vi "FeedbackDecode.vi"() -> ()   [LabVIEW 2020] (continued)
                n758 = Concatenate Strings(w456, ";SS.ExcludeSE=0;" ("EventStr"), w448) -> (w453:string)
                n759 = call "FeedbackDecode_WriteTextEOL.vi"("text"=w453, "refnum in"=w454) -> ()  [unwired: 8 in, 2 out]
                n760 = Bundle By Name(cluster=w460, "EventStr"=w453) -> (w452:T5)
                n761 = call "FeedbackDecode_MLComCtrl.vi"("DecodeClustIn"=w452, "Mode"=T19."SendEvent") -> ()  [unwired: 6 in, 4 out]
              }
              frame True {
                n762 = local read "LoopCnt"() -> (w471:u64)
                n763 = local read "NIPTime"() -> (w465:dbl)
                n764 = Format Into String(w471) -> (resulting string=w461:string)  [unwired: 3 in, 1 out]
                n765 = Concatenate Strings("ExcludeSE:SS.EventID=" ("string"), w461) -> (w470:string)
                n766 = call-poly "FeedbackDecode_VariablesToString.vi"("Format"="%0.0f", "ValueIn"=w465, "FieldName"="NIPTime" ("Key Word")) -> ("StringOut"=w462:string)  [unwired: 4 in]
                n767 = local read "EventParamsFID"() -> (w468:refnum<file>)
                n768 = local read "DecodeClust"() -> (w474:T5)
                n769 = Concatenate Strings(w470, ";SS.ExcludeSE=1;" ("EventStr"), w462) -> (w467:string)
                n770 = call "FeedbackDecode_WriteTextEOL.vi"("text"=w467, "refnum in"=w468) -> ()  [unwired: 8 in, 2 out]
                n771 = Bundle By Name(cluster=w474, "EventStr"=w467) -> (w466:T5)
                n772 = call "FeedbackDecode_MLComCtrl.vi"("DecodeClustIn"=w466, "Mode"=T19."SendEvent") -> ()  [unwired: 6 in, 4 out]
              }
            }
          }
          event Value Change {
            n773 = event-data() -> ("NewVal"=w476:bool)  [unwired: 1 in, 5 out]
            n774 = case shown="True" w476 {
              frame False {
                n775 = local read "LoopCnt"() -> (w487:u64)
                n776 = local read "NIPTime"() -> (w481:dbl)
                n777 = Format Into String(w487) -> (resulting string=w477:string)  [unwired: 3 in, 1 out]
                n778 = Concatenate Strings("StopAcqCAR:SS.EventID=" ("string"), w477) -> (w486:string)
                n779 = local read "EventParamsFID"() -> (w484:refnum<file>)
                n780 = call-poly "FeedbackDecode_VariablesToString.vi"("Format"="%0.0f", "ValueIn"=w481, "FieldName"="NIPTime" ("Key Word")) -> ("StringOut"=w478:string)  [unwired: 4 in]
                n781 = local read "DecodeClust"() -> (w490:T5)
                n782 = Concatenate Strings(w486, ";SS.AcqCAR=0;" ("EventStr"), w478) -> (w483:string)
                n783 = call "FeedbackDecode_WriteTextEOL.vi"("text"=w483, "refnum in"=w484) -> ()  [unwired: 8 in, 2 out]
                n784 = Bundle By Name(cluster=w490, "EventStr"=w483) -> (w482:T5)
                n785 = call "FeedbackDecode_MLComCtrl.vi"("DecodeClustIn"=w482, "Mode"=T19."SendEvent") -> ()  [unwired: 6 in, 4 out]
              }
              frame True {
                n786 = local read "LoopCnt"() -> (w501:u64)
                n787 = local read "NIPTime"() -> (w495:dbl)
                n788 = Format Into String(w501) -> (resulting string=w491:string)  [unwired: 3 in, 1 out]
                n789 = call-poly "FeedbackDecode_VariablesToString.vi"("Format"="%0.0f", "ValueIn"=w495, "FieldName"="NIPTime" ("Key Word")) -> ("StringOut"=w492:string)  [unwired: 4 in]
                n790 = Concatenate Strings("StartAcqCAR:SS.EventID=" ("string"), w491) -> (w500:string)
                n791 = local read "EventParamsFID"() -> (w498:refnum<file>)
                n792 = local read "DecodeClust"() -> (w504:T5)
                n793 = Concatenate Strings(w500, ";SS.AcqCAR=1;" ("EventStr"), w492) -> (w497:string)
                n794 = call "FeedbackDecode_WriteTextEOL.vi"("text"=w497, "refnum in"=w498) -> ()  [unwired: 8 in, 2 out]
                n795 = Bundle By Name(cluster=w504, "EventStr"=w497) -> (w496:T5)
                n796 = call "FeedbackDecode_MLComCtrl.vi"("DecodeClustIn"=w496, "Mode"=T19."SendEvent") -> ()  [unwired: 6 in, 4 out]
              }
            }
          }
          event Value Change {
            n797 = event-data() -> ("NewVal"=w506:bool)  [unwired: 1 in, 5 out]
            n798 = case shown="True" w506 {
              frame False {
              }
              frame True {
                n799 = stacked-sequence {
                  frame #0 {
                    n800 = local read "DecodeClust"() -> (w524:T5)
                    n801 = call "FeedbackDecode_MLComCtrl.vi"("DecodeClustIn"=w524, "Mode"=T19."BuildKalmanStr") -> ("DecodeClustOut"=w523:T5)  [unwired: 6 in, 3 out]
                    n802 = Unbundle By Name(w523) -> ("EventStr"=w531:string, "KalmanType"=w512:T44, "KDFFile"=w516:string)
                    n803 = local read "LoopCnt"() -> (w527:u64)
                    n804 = local read "NIPTime"() -> (w521:dbl)
                    n805 = Format Into String(format string="%s", w512) -> (resulting string=w509:string)  [unwired: 2 in, 1 out]
                    n806 = Format Into String(w527) -> (resulting string=w507:string)  [unwired: 3 in, 1 out]
                    n807 = call-poly "FeedbackDecode_VariablesToString.vi"("ValueIn"=w516, "FieldName"="KDFFile") -> ("StringOut"=w515:string)  [unwired: 5 in]
                    n808 = call-poly "FeedbackDecode_VariablesToString.vi"("Format"="%0.0f", "ValueIn"=w521, "FieldName"="NIPTime" ("Key Word")) -> ("StringOut"=w514:string)  [unwired: 4 in]
                    n809 = Concatenate Strings("ApplyTraining:SS.EventID=" ("string"), w507) -> (w526:string)
                    n810 = Concatenate Strings(w526, ";", w531) -> (w518:string)
                    n811 = local read "EventParamsFID"() -> (w525:refnum<file>)
                    n812 = Bundle By Name(cluster=w523, "EventStr"=w518) -> (w522:T5)
                    n813 = Concatenate Strings(w518, "SS.DecodeType='" ("FieldName"), w509, "';" ("string"), w515, w514) -> (w513:string)
                    n814 = call "FeedbackDecode_WriteTextEOL.vi"("text"=w513, "refnum in"=w525) -> ()  [unwired: 8 in, 2 out]
                    n815 = call "FeedbackDecode_MLComCtrl.vi"("DecodeClustIn"=w522, "Mode"=T19."SendEvent") -> ()  [unwired: 6 in, 4 out]
                  }
                  frame #1 {
                    n816 = property on="KinSrc" class="Enum (strict)"("Val(Sgnl)"=enum16{"Off", "Training", "Decode", "COB"}."Decode" ("Value (Signaling)")) -> ()  [unwired: 2 in, 2 out]
                  }
                }
              }
            }
          }
          event Value Change {
            n817 = event-data() -> ("NewVal"=w534:bool)  [unwired: 1 in, 5 out]
            n818 = case shown="True" w534 {
              frame False {
                n819 = local read "LoopCnt"() -> (w546:u64)
                n820 = local read "NIPTime"() -> (w540:dbl)
                n821 = Format Into String(w546) -> (resulting string=w536:string)  [unwired: 3 in, 1 out]
                n822 = call-poly "FeedbackDecode_VariablesToString.vi"("Format"="%0.0f", "ValueIn"=w540, "FieldName"="NIPTime" ("Key Word")) -> ("StringOut"=w537:string)  [unwired: 4 in]
                n823 = Concatenate Strings("DisableBaseline:SS.EventID=" ("string"), w536) -> (w545:string)
                n824 = local read "EventParamsFID"() -> (w543:refnum<file>)
                n825 = local read "DecodeClust"() -> (w549:T5)
                n826 = Concatenate Strings(w545, ";SS.ApplyBaseline=0;" ("EventStr"), w537) -> (w542:string)
                n827 = call "FeedbackDecode_WriteTextEOL.vi"("text"=w542, "refnum in"=w543) -> ()  [unwired: 8 in, 2 out]
                n828 = Bundle By Name(cluster=w549, "EventStr"=w542) -> (w541:T5)
                n829 = call "FeedbackDecode_MLComCtrl.vi"("DecodeClustIn"=w541, "Mode"=T19."SendEvent") -> ()  [unwired: 6 in, 4 out]
              }
              frame True {
                n830 = local read "LoopCnt"() -> (w560:u64)
                n831 = local read "NIPTime"() -> (w554:dbl)
                n832 = Format Into String(w560) -> (resulting string=w550:string)  [unwired: 3 in, 1 out]
                n833 = Concatenate Strings("EnableBaseline:SS.EventID=" ("string"), w550) -> (w559:string)
                n834 = local read "EventParamsFID"() -> (w557:refnum<file>)
                n835 = call-poly "FeedbackDecode_VariablesToString.vi"("Format"="%0.0f", "ValueIn"=w554, "FieldName"="NIPTime" ("Key Word")) -> ("StringOut"=w551:string)  [unwired: 4 in]
                n836 = local read "DecodeClust"() -> (w563:T5)
                n837 = Concatenate Strings(w559, ";SS.ApplyBaseline=1;" ("EventStr"), w551) -> (w556:string)
                n838 = call "FeedbackDecode_WriteTextEOL.vi"("text"=w556, "refnum in"=w557) -> ()  [unwired: 8 in, 2 out]
                n839 = Bundle By Name(cluster=w563, "EventStr"=w556) -> (w555:T5)
                n840 = call "FeedbackDecode_MLComCtrl.vi"("DecodeClustIn"=w555, "Mode"=T19."SendEvent") -> ()  [unwired: 6 in, 4 out]
              }
            }
          }
          event Value Change {
            n841 = event-data() -> ("NewVal"=w564:bool)  [unwired: 1 in, 5 out]
            n842 = case shown="True" w564 {
              frame False {
                n843 = disable-structure shown="Disabled" {
                  frame Disabled {
                    n844 = local read "LoopCnt"() -> (w576:u64)
                    n845 = local read "NIPTime"() -> (w570:dbl)
                    n846 = Format Into String(w576) -> (resulting string=w566:string)  [unwired: 3 in, 1 out]
                    n847 = call-poly "FeedbackDecode_VariablesToString.vi"("Format"="%0.0f", "ValueIn"=w570, "FieldName"="NIPTime" ("Key Word")) -> ("StringOut"=w567:string)  [unwired: 4 in]
                    n848 = Concatenate Strings("DisableBaseline:SS.EventID=" ("string"), w566) -> (w575:string)
                    n849 = local read "EventParamsFID"() -> (w573:refnum<file>)
                    n850 = local read "DecodeClust"() -> (w579:T5)
                    n851 = Concatenate Strings(w575, ";SS.ApplyBaseline=0;" ("EventStr"), w567) -> (w572:string)
                    n852 = call "FeedbackDecode_WriteTextEOL.vi"("text"=w572, "refnum in"=w573) -> ()  [unwired: 8 in, 2 out]
                    n853 = Bundle By Name(cluster=w579, "EventStr"=w572) -> (w571:T5)
                    n854 = call "FeedbackDecode_MLComCtrl.vi"("DecodeClustIn"=w571, "Mode"=T19."SendEvent") -> ()  [unwired: 6 in, 4 out]
                  }
                  frame Enabled {
                  }
                }
              }
              frame True {
                n855 = local read "LoopCnt"() -> (w590:u64)
                n856 = local read "NIPTime"() -> (w584:dbl)
                n857 = Format Into String(w590) -> (resulting string=w580:string)  [unwired: 3 in, 1 out]
                n858 = Concatenate Strings("ExportTraining:SS.EventID=" ("string"), w580) -> (w589:string)
                n859 = local read "EventParamsFID"() -> (w587:refnum<file>)
                n860 = call-poly "FeedbackDecode_VariablesToString.vi"("Format"="%0.0f", "ValueIn"=w584, "FieldName"="NIPTime" ("Key Word")) -> ("StringOut"=w581:string)  [unwired: 4 in]
                n861 = local read "DecodeClust"() -> (w593:T5)
                n862 = Concatenate Strings(w589, ";SS.ExportTraining=1;" ("EventStr"), w581) -> (w586:string)
                n863 = call "FeedbackDecode_WriteTextEOL.vi"("text"=w586, "refnum in"=w587) -> ()  [unwired: 8 in, 2 out]
                n864 = Bundle By Name(cluster=w593, "EventStr"=w586) -> (w585:T5)
                n865 = call "FeedbackDecode_MLComCtrl.vi"("DecodeClustIn"=w585, "Mode"=T19."SendEvent") -> ()  [unwired: 6 in, 4 out]
              }
            }
          }
          event Value Change {
            n866 = event-data() -> ("NewVal"=w594:bool)  [unwired: 1 in, 5 out]
            n867 = case shown="True" w594 {
              frame False {
                n868 = local read "LoopCnt"() -> (w606:u64)
                n869 = local read "NIPTime"() -> (w600:dbl)
                n870 = Format Into String(w606) -> (resulting string=w596:string)  [unwired: 3 in, 1 out]
                n871 = call-poly "FeedbackDecode_VariablesToString.vi"("Format"="%0.0f", "ValueIn"=w600, "FieldName"="NIPTime" ("Key Word")) -> ("StringOut"=w597:string)  [unwired: 4 in]
                n872 = Concatenate Strings("LatchingFilter:SS.EventID=" ("string"), w596) -> (w605:string)
                n873 = local read "EventParamsFID"() -> (w603:refnum<file>)
                n874 = local read "DecodeClust"() -> (w609:T5)
                n875 = Concatenate Strings(w605, ";SS.LatchingFilter=0;" ("EventStr"), w597) -> (w602:string)
                n876 = call "FeedbackDecode_WriteTextEOL.vi"("text"=w602, "refnum in"=w603) -> ()  [unwired: 8 in, 2 out]
                n877 = Bundle By Name(cluster=w609, "EventStr"=w602) -> (w601:T5)
                n878 = call "FeedbackDecode_MLComCtrl.vi"("DecodeClustIn"=w601, "Mode"=T19."SendEvent") -> ()  [unwired: 6 in, 4 out]
              }
              frame True {
                n879 = local read "LoopCnt"() -> (w620:u64)
                n880 = local read "NIPTime"() -> (w614:dbl)
                n881 = Format Into String(w620) -> (resulting string=w610:string)  [unwired: 3 in, 1 out]
                n882 = Concatenate Strings("LatchingFilter:SS.EventID=" ("string"), w610) -> (w619:string)
                n883 = local read "EventParamsFID"() -> (w617:refnum<file>)
                n884 = call-poly "FeedbackDecode_VariablesToString.vi"("Format"="%0.0f", "ValueIn"=w614, "FieldName"="NIPTime" ("Key Word")) -> ("StringOut"=w611:string)  [unwired: 4 in]
                n885 = local read "DecodeClust"() -> (w623:T5)
                n886 = Concatenate Strings(w619, ";SS.LatchingFilter=1;" ("EventStr"), w611) -> (w616:string)
                n887 = call "FeedbackDecode_WriteTextEOL.vi"("text"=w616, "refnum in"=w617) -> ()  [unwired: 8 in, 2 out]
                n888 = Bundle By Name(cluster=w623, "EventStr"=w616) -> (w615:T5)
                n889 = call "FeedbackDecode_MLComCtrl.vi"("DecodeClustIn"=w615, "Mode"=T19."SendEvent") -> ()  [unwired: 6 in, 4 out]
              }
            }
          }
          event Value Change {
            n890 = event-data() -> ("NewVal"=w624:bool)  [unwired: 1 in, 5 out]
            n891 = case shown="True" w624 {
              frame False {
                n892 = local read "LoopCnt"() -> (w636:u64)
                n893 = local read "NIPTime"() -> (w630:dbl)
                n894 = Format Into String(w636) -> (resulting string=w626:string)  [unwired: 3 in, 1 out]
                n895 = call-poly "FeedbackDecode_VariablesToString.vi"("Format"="%0.0f", "ValueIn"=w630, "FieldName"="NIPTime" ("Key Word")) -> ("StringOut"=w627:string)  [unwired: 4 in]
                n896 = Concatenate Strings("EEGTrigger:SS.EventID=" ("string"), w626) -> (w635:string)
                n897 = local read "EventParamsFID"() -> (w633:refnum<file>)
                n898 = local read "DecodeClust"() -> (w639:T5)
                n899 = Concatenate Strings(w635, ";SS.EEGTrigger=0;" ("EventStr"), w627) -> (w632:string)
                n900 = call "FeedbackDecode_WriteTextEOL.vi"("text"=w632, "refnum in"=w633) -> ()  [unwired: 8 in, 2 out]
                n901 = Bundle By Name(cluster=w639, "EventStr"=w632) -> (w631:T5)
                n902 = call "FeedbackDecode_MLComCtrl.vi"("DecodeClustIn"=w631, "Mode"=T19."SendEvent") -> ()  [unwired: 6 in, 4 out]
              }
              frame True {
                n903 = local read "LoopCnt"() -> (w650:u64)
                n904 = local read "NIPTime"() -> (w644:dbl)
                n905 = Format Into String(w650) -> (resulting string=w640:string)  [unwired: 3 in, 1 out]
                n906 = Concatenate Strings("EEGTrigger:SS.EventID=" ("string"), w640) -> (w649:string)
                n907 = local read "EventParamsFID"() -> (w647:refnum<file>)
                n908 = call-poly "FeedbackDecode_VariablesToString.vi"("Format"="%0.0f", "ValueIn"=w644, "FieldName"="NIPTime" ("Key Word")) -> ("StringOut"=w641:string)  [unwired: 4 in]
                n909 = local read "DecodeClust"() -> (w653:T5)
                n910 = Concatenate Strings(w649, ";SS.EEGTrigger=1;" ("EventStr"), w641) -> (w646:string)
                n911 = call "FeedbackDecode_WriteTextEOL.vi"("text"=w646, "refnum in"=w647) -> ()  [unwired: 8 in, 2 out]
                n912 = Bundle By Name(cluster=w653, "EventStr"=w646) -> (w645:T5)
                n913 = call "FeedbackDecode_MLComCtrl.vi"("DecodeClustIn"=w645, "Mode"=T19."SendEvent") -> ()  [unwired: 6 in, 4 out]
              }
            }
          }
          event Value Change {
            n914 = event-data() -> ("NewVal"=w654:bool)  [unwired: 1 in, 5 out]
            n915 = case shown="True" w654 {
              frame False {
                n916 = local read "LoopCnt"() -> (w666:u64)
                n917 = local read "NIPTime"() -> (w660:dbl)
                n918 = Format Into String(w666) -> (resulting string=w656:string)  [unwired: 3 in, 1 out]
                n919 = call-poly "FeedbackDecode_VariablesToString.vi"("Format"="%0.0f", "ValueIn"=w660, "FieldName"="NIPTime" ("Key Word")) -> ("StringOut"=w657:string)  [unwired: 4 in]
                n920 = Concatenate Strings("ConnectECG:SS.EventID=" ("string"), w656) -> (w665:string)
                n921 = local read "EventParamsFID"() -> (w663:refnum<file>)
                n922 = local read "DecodeClust"() -> (w669:T5)
                n923 = Concatenate Strings(w665, ";SS.ConnectECG=0;" ("EventStr"), w657) -> (w662:string)
                n924 = call "FeedbackDecode_WriteTextEOL.vi"("text"=w662, "refnum in"=w663) -> ()  [unwired: 8 in, 2 out]
                n925 = Bundle By Name(cluster=w669, "EventStr"=w662) -> (w661:T5)
                n926 = call "FeedbackDecode_MLComCtrl.vi"("DecodeClustIn"=w661, "Mode"=T19."SendEvent") -> ()  [unwired: 6 in, 4 out]
              }
              frame True {
                n927 = local read "LoopCnt"() -> (w680:u64)
                n928 = local read "NIPTime"() -> (w674:dbl)
                n929 = Format Into String(w680) -> (resulting string=w670:string)  [unwired: 3 in, 1 out]
                n930 = Concatenate Strings("ConnectECG:SS.EventID=" ("string"), w670) -> (w679:string)
                n931 = local read "EventParamsFID"() -> (w677:refnum<file>)
                n932 = call-poly "FeedbackDecode_VariablesToString.vi"("Format"="%0.0f", "ValueIn"=w674, "FieldName"="NIPTime" ("Key Word")) -> ("StringOut"=w671:string)  [unwired: 4 in]
                n933 = local read "DecodeClust"() -> (w683:T5)
                n934 = Concatenate Strings(w679, ";SS.ConnectECG=1;" ("EventStr"), w671) -> (w676:string)
                n935 = call "FeedbackDecode_WriteTextEOL.vi"("text"=w676, "refnum in"=w677) -> ()  [unwired: 8 in, 2 out]
                n936 = Bundle By Name(cluster=w683, "EventStr"=w676) -> (w675:T5)
                n937 = call "FeedbackDecode_MLComCtrl.vi"("DecodeClustIn"=w675, "Mode"=T19."SendEvent") -> ()  [unwired: 6 in, 4 out]
              }
            }
          }
          event Value Change {
            n938 = event-data() -> ("NewVal"=w684:bool)  [unwired: 1 in, 5 out]
            n939 = case shown="False" w684 {
              frame False {
                n940 = local read "LoopCnt"() -> (w696:u64)
                n941 = local read "NIPTime"() -> (w690:dbl)
                n942 = Format Into String(w696) -> (resulting string=w686:string)  [unwired: 3 in, 1 out]
                n943 = call-poly "FeedbackDecode_VariablesToString.vi"("Format"="%0.0f", "ValueIn"=w690, "FieldName"="NIPTime" ("Key Word")) -> ("StringOut"=w687:string)  [unwired: 4 in]
                n944 = Concatenate Strings("ConnectIMU:SS.EventID=" ("string"), w686) -> (w695:string)
                n945 = local read "EventParamsFID"() -> (w693:refnum<file>)
                n946 = local read "DecodeClust"() -> (w699:T5)
                n947 = Concatenate Strings(w695, ";SS.ConnectIMU=0;" ("EventStr"), w687) -> (w692:string)
                n948 = call "FeedbackDecode_WriteTextEOL.vi"("text"=w692, "refnum in"=w693) -> ()  [unwired: 8 in, 2 out]
                n949 = Bundle By Name(cluster=w699, "EventStr"=w692) -> (w691:T5)
                n950 = call "FeedbackDecode_MLComCtrl.vi"("DecodeClustIn"=w691, "Mode"=T19."SendEvent") -> ()  [unwired: 6 in, 4 out]
              }
              frame True {
                n951 = local read "LoopCnt"() -> (w710:u64)
                n952 = local read "NIPTime"() -> (w704:dbl)
                n953 = Format Into String(w710) -> (resulting string=w700:string)  [unwired: 3 in, 1 out]
                n954 = Concatenate Strings("ConnectIMU:SS.EventID=" ("string"), w700) -> (w709:string)
                n955 = local read "EventParamsFID"() -> (w707:refnum<file>)
                n956 = call-poly "FeedbackDecode_VariablesToString.vi"("Format"="%0.0f", "ValueIn"=w704, "FieldName"="NIPTime" ("Key Word")) -> ("StringOut"=w701:string)  [unwired: 4 in]
                n957 = local read "DecodeClust"() -> (w713:T5)
                n958 = Concatenate Strings(w709, ";SS.ConnectIMU=1;" ("EventStr"), w701) -> (w706:string)
                n959 = call "FeedbackDecode_WriteTextEOL.vi"("text"=w706, "refnum in"=w707) -> ()  [unwired: 8 in, 2 out]
                n960 = Bundle By Name(cluster=w713, "EventStr"=w706) -> (w705:T5)
                n961 = call "FeedbackDecode_MLComCtrl.vi"("DecodeClustIn"=w705, "Mode"=T19."SendEvent") -> ()  [unwired: 6 in, 4 out]
              }
            }
          }
          event Value Change {
            n962 = event-data() -> ("NewVal"=w714:bool)  [unwired: 1 in, 5 out]
            n963 = case shown="True" w714 {
              frame False {
                n964 = local read "LoopCnt"() -> (w726:u64)
                n965 = local read "NIPTime"() -> (w720:dbl)
                n966 = Format Into String(w726) -> (resulting string=w716:string)  [unwired: 3 in, 1 out]
                n967 = call-poly "FeedbackDecode_VariablesToString.vi"("Format"="%0.0f", "ValueIn"=w720, "FieldName"="NIPTime" ("Key Word")) -> ("StringOut"=w717:string)  [unwired: 4 in]
                n968 = Concatenate Strings("ECGTriggerTargets:SS.EventID=" ("string"), w716) -> (w725:string)
                n969 = local read "EventParamsFID"() -> (w723:refnum<file>)
                n970 = local read "DecodeClust"() -> (w729:T5)
                n971 = Concatenate Strings(w725, ";SS.ECGTriggerTargets=0;" ("EventStr"), w717) -> (w722:string)
                n972 = call "FeedbackDecode_WriteTextEOL.vi"("text"=w722, "refnum in"=w723) -> ()  [unwired: 8 in, 2 out]
                n973 = Bundle By Name(cluster=w729, "EventStr"=w722) -> (w721:T5)
                n974 = call "FeedbackDecode_MLComCtrl.vi"("DecodeClustIn"=w721, "Mode"=T19."SendEvent") -> ()  [unwired: 6 in, 4 out]
              }
              frame True {
                n975 = local read "LoopCnt"() -> (w740:u64)
                n976 = local read "NIPTime"() -> (w734:dbl)
                n977 = Format Into String(w740) -> (resulting string=w730:string)  [unwired: 3 in, 1 out]
                n978 = Concatenate Strings("ECGTriggerTargets:SS.EventID=" ("string"), w730) -> (w739:string)
                n979 = local read "EventParamsFID"() -> (w737:refnum<file>)
                n980 = call-poly "FeedbackDecode_VariablesToString.vi"("Format"="%0.0f", "ValueIn"=w734, "FieldName"="NIPTime" ("Key Word")) -> ("StringOut"=w731:string)  [unwired: 4 in]
                n981 = local read "DecodeClust"() -> (w743:T5)
                n982 = Concatenate Strings(w739, ";SS.ECGTriggerTargets=1;" ("EventStr"), w731) -> (w736:string)
                n983 = call "FeedbackDecode_WriteTextEOL.vi"("text"=w736, "refnum in"=w737) -> ()  [unwired: 8 in, 2 out]
                n984 = Bundle By Name(cluster=w743, "EventStr"=w736) -> (w735:T5)
                n985 = call "FeedbackDecode_MLComCtrl.vi"("DecodeClustIn"=w735, "Mode"=T19."SendEvent") -> ()  [unwired: 6 in, 4 out]
              }
            }
          }
          event Value Change {
            n986 = event-data() -> ("NewVal"=w744:bool)  [unwired: 1 in, 5 out]
            n987 = case shown="False" w744 {
              frame False {
                n988 = local read "LoopCnt"() -> (w756:u64)
                n989 = local read "NIPTime"() -> (w750:dbl)
                n990 = Format Into String(w756) -> (resulting string=w746:string)  [unwired: 3 in, 1 out]
                n991 = call-poly "FeedbackDecode_VariablesToString.vi"("Format"="%0.0f", "ValueIn"=w750, "FieldName"="NIPTime" ("Key Word")) -> ("StringOut"=w747:string)  [unwired: 4 in]
                n992 = Concatenate Strings("RecordIMUwithTraining:SS.EventID=" ("string"), w746) -> (w755:string)
                n993 = local read "EventParamsFID"() -> (w753:refnum<file>)
                n994 = local read "DecodeClust"() -> (w759:T5)
                n995 = Concatenate Strings(w755, ";SS.RecordIMUwithTraining=0;" ("EventStr"), w747) -> (w752:string)
                n996 = call "FeedbackDecode_WriteTextEOL.vi"("text"=w752, "refnum in"=w753) -> ()  [unwired: 8 in, 2 out]
                n997 = Bundle By Name(cluster=w759, "EventStr"=w752) -> (w751:T5)
                n998 = call "FeedbackDecode_MLComCtrl.vi"("DecodeClustIn"=w751, "Mode"=T19."SendEvent") -> ()  [unwired: 6 in, 4 out]
              }
              frame True {
                n999 = local read "LoopCnt"() -> (w770:u64)
                n1000 = local read "NIPTime"() -> (w764:dbl)
                n1001 = Format Into String(w770) -> (resulting string=w760:string)  [unwired: 3 in, 1 out]
                n1002 = Concatenate Strings("RecordIMUwithTraining:SS.EventID=" ("string"), w760) -> (w769:string)
                n1003 = local read "EventParamsFID"() -> (w767:refnum<file>)
                n1004 = call-poly "FeedbackDecode_VariablesToString.vi"("Format"="%0.0f", "ValueIn"=w764, "FieldName"="NIPTime" ("Key Word")) -> ("StringOut"=w761:string)  [unwired: 4 in]
                n1005 = local read "DecodeClust"() -> (w773:T5)
                n1006 = Concatenate Strings(w769, ";SS.RecordIMUwithTraining=1;" ("EventStr"), w761) -> (w766:string)
                n1007 = call "FeedbackDecode_WriteTextEOL.vi"("text"=w766, "refnum in"=w767) -> ()  [unwired: 8 in, 2 out]
                n1008 = Bundle By Name(cluster=w773, "EventStr"=w766) -> (w765:T5)
                n1009 = call "FeedbackDecode_MLComCtrl.vi"("DecodeClustIn"=w765, "Mode"=T19."SendEvent") -> ()  [unwired: 6 in, 4 out]
              }
            }
          }
          event Value Change {
            n1010 = event-data() -> ("NewVal"=w774:bool)  [unwired: 1 in, 5 out]
            n1011 = case shown="True" w774 {
              frame False {
                n1012 = local read "LoopCnt"() -> (w786:u64)
                n1013 = local read "NIPTime"() -> (w780:dbl)
                n1014 = Format Into String(w786) -> (resulting string=w776:string)  [unwired: 3 in, 1 out]
                n1015 = call-poly "FeedbackDecode_VariablesToString.vi"("Format"="%0.0f", "ValueIn"=w780, "FieldName"="NIPTime" ("Key Word")) -> ("StringOut"=w777:string)  [unwired: 4 in]
                n1016 = Concatenate Strings("SecondaryTask:SS.EventID=" ("string"), w776) -> (w785:string)
                n1017 = local read "EventParamsFID"() -> (w783:refnum<file>)
                n1018 = local read "DecodeClust"() -> (w789:T5)
                n1019 = Concatenate Strings(w785, ";SS.SecondaryTask=0;" ("EventStr"), w777) -> (w782:string)
                n1020 = call "FeedbackDecode_WriteTextEOL.vi"("text"=w782, "refnum in"=w783) -> ()  [unwired: 8 in, 2 out]
                n1021 = Bundle By Name(cluster=w789, "EventStr"=w782) -> (w781:T5)
                n1022 = call "FeedbackDecode_MLComCtrl.vi"("DecodeClustIn"=w781, "Mode"=T19."SendEvent") -> ()  [unwired: 6 in, 4 out]
              }
              frame True {
                n1023 = local read "LoopCnt"() -> (w800:u64)
                n1024 = local read "NIPTime"() -> (w794:dbl)
                n1025 = Format Into String(w800) -> (resulting string=w790:string)  [unwired: 3 in, 1 out]
                n1026 = Concatenate Strings("SecondaryTask:SS.EventID=" ("string"), w790) -> (w799:string)
                n1027 = local read "EventParamsFID"() -> (w797:refnum<file>)
                n1028 = call-poly "FeedbackDecode_VariablesToString.vi"("Format"="%0.0f", "ValueIn"=w794, "FieldName"="NIPTime" ("Key Word")) -> ("StringOut"=w791:string)  [unwired: 4 in]
                n1029 = local read "DecodeClust"() -> (w803:T5)
                n1030 = Concatenate Strings(w799, ";SS.SecondaryTask=1;" ("EventStr"), w791) -> (w796:string)
                n1031 = call "FeedbackDecode_WriteTextEOL.vi"("text"=w796, "refnum in"=w797) -> ()  [unwired: 8 in, 2 out]
                n1032 = Bundle By Name(cluster=w803, "EventStr"=w796) -> (w795:T5)
                n1033 = call "FeedbackDecode_MLComCtrl.vi"("DecodeClustIn"=w795, "Mode"=T19."SendEvent") -> ()  [unwired: 6 in, 4 out]
              }
            }
          }
          event Value Change {
            n1034 = event-data() -> ("NewVal"=w807:dbl)  [unwired: 1 in, 5 out]
            n1035 = local read "LoopCnt"() -> (w811:u64)
            n1036 = local read "NIPTime"() -> (w816:dbl)
            n1037 = Format Into String(w811) -> (resulting string=w819:string)  [unwired: 3 in, 1 out]
            n1038 = call-poly "FeedbackDecode_VariablesToString.vi"("Format"="%0.0f" ("EventStr"), "ValueIn"=w807, "FieldName"="SecondaryTaskMinBetweenStim" ("EventStr")) -> ("StringOut"=w805:string)  [unwired: 4 in]
            n1039 = Concatenate Strings("SecondaryTaskMinBetweenStim:SS.EventID=" ("string"), w819) -> (w812:string)
            n1040 = local read "EventParamsFID"() -> (w813:refnum<file>)
            n1041 = call-poly "FeedbackDecode_VariablesToString.vi"("Format"="%0.0f", "ValueIn"=w816, "FieldName"="NIPTime" ("Key Word")) -> ("StringOut"=w806:string)  [unwired: 4 in]
            n1042 = local read "DecodeClust"() -> (w808:T5)
            n1043 = Concatenate Strings(w812, ";" ("EventStr"), w805, w806) -> (w814:string)
            n1044 = call "FeedbackDecode_WriteTextEOL.vi"("text"=w814, "refnum in"=w813) -> ()  [unwired: 8 in, 2 out]
            n1045 = Bundle By Name(cluster=w808, "EventStr"=w814) -> (w815:T5)
            n1046 = call "FeedbackDecode_MLComCtrl.vi"("DecodeClustIn"=w815, "Mode"=T19."SendEvent") -> ()  [unwired: 6 in, 4 out]
          }
          event Value Change {
            n1047 = event-data() -> ("NewVal"=w825:dbl)  [unwired: 1 in, 5 out]
            n1048 = local read "LoopCnt"() -> (w832:u64)
            n1049 = call-poly "FeedbackDecode_VariablesToString.vi"("Format"="%0.0f" ("EventStr"), "ValueIn"=w825, "FieldName"="SecondaryTaskVarBetweenStim" ("EventStr")) -> ("StringOut"=w824:string)  [unwired: 4 in]
            n1050 = local read "NIPTime"() -> (w837:dbl)
            n1051 = Format Into String(w832) -> (resulting string=w840:string)  [unwired: 3 in, 1 out]
            n1052 = Concatenate Strings("SecondaryTaskVarBetweenStim:SS.EventID=" ("string"), w840) -> (w833:string)
            n1053 = local read "EventParamsFID"() -> (w834:refnum<file>)
            n1054 = call-poly "FeedbackDecode_VariablesToString.vi"("Format"="%0.0f", "ValueIn"=w837, "FieldName"="NIPTime" ("Key Word")) -> ("StringOut"=w823:string)  [unwired: 4 in]
            n1055 = local read "DecodeClust"() -> (w829:T5)
            n1056 = Concatenate Strings(w833, ";" ("EventStr"), w824, w823) -> (w835:string)
            n1057 = call "FeedbackDecode_WriteTextEOL.vi"("text"=w835, "refnum in"=w834) -> ()  [unwired: 8 in, 2 out]
            n1058 = Bundle By Name(cluster=w829, "EventStr"=w835) -> (w836:T5)
            n1059 = call "FeedbackDecode_MLComCtrl.vi"("DecodeClustIn"=w836, "Mode"=T19."SendEvent") -> ()  [unwired: 6 in, 4 out]
          }
          event Value Change {
            n1060 = event-data() -> ("NewVal"=w844:dbl)  [unwired: 1 in, 5 out]
            n1061 = local read "LoopCnt"() -> (w851:u64)
            n1062 = local read "NIPTime"() -> (w856:dbl)
            n1063 = Format Into String(w851) -> (resulting string=w859:string)  [unwired: 3 in, 1 out]
            n1064 = call-poly "FeedbackDecode_VariablesToString.vi"("Format"="%0.0f" ("EventStr"), "ValueIn"=w844, "FieldName"="SecondaryTaskStimDur" ("EventStr")) -> ("StringOut"=w843:string)  [unwired: 4 in]
            n1065 = Concatenate Strings("SecondaryTaskStimDur:SS.EventID=" ("string"), w859) -> (w852:string)
            n1066 = local read "EventParamsFID"() -> (w853:refnum<file>)
            n1067 = call-poly "FeedbackDecode_VariablesToString.vi"("Format"="%0.0f", "ValueIn"=w856, "FieldName"="NIPTime" ("Key Word")) -> ("StringOut"=w842:string)  [unwired: 4 in]
            n1068 = local read "DecodeClust"() -> (w848:T5)
            n1069 = Concatenate Strings(w852, ";" ("EventStr"), w843, w842) -> (w854:string)
            n1070 = call "FeedbackDecode_WriteTextEOL.vi"("text"=w854, "refnum in"=w853) -> ()  [unwired: 8 in, 2 out]
            n1071 = Bundle By Name(cluster=w848, "EventStr"=w854) -> (w855:T5)
            n1072 = call "FeedbackDecode_MLComCtrl.vi"("DecodeClustIn"=w855, "Mode"=T19."SendEvent") -> ()  [unwired: 6 in, 4 out]
          }
          event Value Change {
            n1073 = event-data() -> ("NewVal"=w861:bool)  [unwired: 1 in, 5 out]
            n1074 = case shown="True" w861 {
              frame False {
                n1075 = local read "LoopCnt"() -> (w873:u64)
                n1076 = local read "NIPTime"() -> (w867:dbl)
                n1077 = Format Into String(w873) -> (resulting string=w863:string)  [unwired: 3 in, 1 out]
                n1078 = Concatenate Strings("DisableCAR:SS.EventID=" ("string"), w863) -> (w872:string)
                n1079 = local read "EventParamsFID"() -> (w870:refnum<file>)
                n1080 = call-poly "FeedbackDecode_VariablesToString.vi"("Format"="%0.0f", "ValueIn"=w867, "FieldName"="NIPTime" ("Key Word")) -> ("StringOut"=w864:string)  [unwired: 4 in]
                n1081 = local read "DecodeClust"() -> (w876:T5)
                n1082 = Concatenate Strings(w872, ";SS.CAR=0;" ("EventStr"), w864) -> (w869:string)
                n1083 = call "FeedbackDecode_WriteTextEOL.vi"("text"=w869, "refnum in"=w870) -> ()  [unwired: 8 in, 2 out]
                n1084 = Bundle By Name(cluster=w876, "EventStr"=w869) -> (w868:T5)
                n1085 = call "FeedbackDecode_MLComCtrl.vi"("DecodeClustIn"=w868, "Mode"=T19."SendEvent") -> ()  [unwired: 6 in, 4 out]
              }
              frame True {
                n1086 = local read "DecodeClust"() -> (w883:T5)
                n1087 = local read "NIPTime"() -> (w881:dbl)
                n1088 = Unbundle By Name(w883) -> ("BadUEAElects"=w892:dbl[])
                n1089 = local read "LoopCnt"() -> (w889:u64)
                n1090 = call-poly "FeedbackDecode_VariablesToString.vi"("Format"="%0.0f", "ValueIn"=w881, "FieldName"="NIPTime" ("Key Word")) -> ("StringOut"=w878:string)  [unwired: 4 in]
                n1091 = Format Into String(w889) -> (resulting string=w877:string)  [unwired: 3 in, 1 out]
                n1092 = Concatenate Strings("EnableCAR:SS.EventID=" ("string"), w877) -> (w888:string)
                n1093 = call-poly "FeedbackDecode_VariablesToString.vi"("ValueIn"=w892, "FieldName"="BadUEAElects") -> ("StringOut"=w884:string)  [unwired: 5 in]
                n1094 = local read "EventParamsFID"() -> (w886:refnum<file>)
                n1095 = Concatenate Strings(w888, ";SS.CAR=1;" ("EventStr"), w884, w878) -> (w885:string)
                n1096 = call "FeedbackDecode_WriteTextEOL.vi"("text"=w885, "refnum in"=w886) -> ()  [unwired: 8 in, 2 out]
                n1097 = Bundle By Name(cluster=w883, "EventStr"=w885) -> (w882:T5)
                n1098 = call "FeedbackDecode_MLComCtrl.vi"("DecodeClustIn"=w882, "Mode"=T19."SendEvent") -> ()  [unwired: 6 in, 4 out]
              }
            }
          }
          event Value Change {
            n1099 = event-data() -> ("NewVal"=w894:bool)  [unwired: 1 in, 5 out]
            n1100 = case shown="True" w894 {
              frame False {
              }
              frame True {
                n1101 = local read "DecodeClust"() -> (w902:T5)
                n1102 = local read "DecodeClust"() -> (w917:T5)
                n1103 = Bundle By Name(cluster=w917, "CtrlButtons.DEKARestart"=FALSE) -> (w916:T5)
                n1104 = Unbundle By Name(w902) -> ("*Prosthesis"=w901:enum16{"MaleRight", "MaleLeft"})
                n1105 = local write "DecodeClust"(w916) -> ()
                n1106 = local read "LoopCnt"() -> (w912:u64)
                n1107 = local read "NIPTime"() -> (w907:dbl)
                n1108 = Format Into String(w901) -> (resulting string=w900:string)  [unwired: 3 in, 1 out]
                n1109 = Format Into String(w912) -> (resulting string=w904:string)  [unwired: 3 in, 1 out]
                n1110 = Concatenate Strings("RestartDEKA:SS.EventID=" ("string"), w904, ";" ("string")) -> (w911:string)
                n1111 = Concatenate Strings("SS.Prosthesis='" ("EventStr"), w900, "';" ("string")) -> (w896:string)
                n1112 = call-poly "FeedbackDecode_VariablesToString.vi"("Format"="%0.0f", "ValueIn"=w907, "FieldName"="NIPTime" ("Key Word")) -> ("StringOut"=w897:string)  [unwired: 4 in]
                n1113 = global write "FeedbackDecode_Globals.vi" "FD_DEKARestart"(TRUE ("G_DEKARestart")) -> ()
                n1114 = local read "EventParamsFID"() -> (w910:refnum<file>)
                n1115 = Concatenate Strings(w911, w896, w897) -> (w909:string)
                n1116 = call "FeedbackDecode_WriteTextEOL.vi"("text"=w909, "refnum in"=w910) -> ()  [unwired: 8 in, 2 out]
                n1117 = Bundle By Name(cluster=w902, "EventStr"=w909) -> (w908:T5)
                n1118 = call "FeedbackDecode_MLComCtrl.vi"("DecodeClustIn"=w908, "Mode"=T19."SendEvent") -> ()  [unwired: 6 in, 4 out]
              }
            }
          }
          event Value Change {
            n1119 = event-data() -> ("NewVal"=w919:bool)  [unwired: 1 in, 5 out]
            n1120 = case shown="True" w919 {
              frame False {
              }
              frame True {
                n1121 = local read "DecodeClust"() -> (w937:T5)
                n1122 = Bundle By Name(cluster=w937, "CtrlButtons.CalDEKA"=FALSE ("CtrlButtons.DEKARestart")) -> (w936:T5)
                n1123 = local read "LoopCnt"() -> (w931:u64)
                n1124 = local write "DecodeClust"(w936) -> ()
                n1125 = local read "NIPTime"() -> (w926:dbl)
                n1126 = Format Into String(w931) -> (resulting string=w923:string)  [unwired: 3 in, 1 out]
                n1127 = Concatenate Strings("CalibrateDEKA:SS.EventID=" ("string"), w923, ";" ("string")) -> (w930:string)
                n1128 = call-poly "FeedbackDecode_VariablesToString.vi"("Format"="%0.0f", "ValueIn"=w926, "FieldName"="NIPTime" ("Key Word")) -> ("StringOut"=w922:string)  [unwired: 4 in]
                n1129 = local read "EventParamsFID"() -> (w929:refnum<file>)
                n1130 = local read "DecodeClust"() -> (w934:T5)
                n1131 = Concatenate Strings(w930, w922) -> (w928:string)
                n1132 = call "FeedbackDecode_WriteTextEOL.vi"("text"=w928, "refnum in"=w929) -> ()  [unwired: 8 in, 2 out]
                n1133 = Bundle By Name(cluster=w934, "EventStr"=w928) -> (w927:T5)
                n1134 = call "FeedbackDecode_MLComCtrl.vi"("DecodeClustIn"=w927, "Mode"=T19."SendEvent") -> ()  [unwired: 6 in, 4 out]
              }
            }
          }
          event Value Change {
            n1135 = event-data() -> ("NewVal"=w956:bool)  [unwired: 1 in, 5 out]
            n1136 = case shown="True" w956 {
              tunnel: [0.0 1.0] -> w940
              frame False {
              }
              frame True {
                n1137 = local read "DecodeClust"() -> (w962:T5)
                n1138 = Bundle By Name(cluster=w962, "CtrlButtons.CalDEKA"=FALSE ("CtrlButtons.DEKARestart")) -> (w961:T5)
                n1139 = local write "DecodeClust"(w961) -> ()
              }
            }
            n1140 = call-poly "FeedbackDecode_VariablesToString.vi"("Format"="%d", "ValueIn"=w940, "FieldName"="DEKA.Ready" ("string")) -> ("StringOut"=w938:string)  [unwired: 4 in]
            n1141 = local read "LoopCnt"() -> (w952:u64)
            n1142 = local read "NIPTime"() -> (w947:dbl)
            n1143 = Format Into String(w952) -> (resulting string=w944:string)  [unwired: 3 in, 1 out]
            n1144 = Concatenate Strings("ConnectDEKA:SS.EventID=" ("string"), w944, ";" ("string")) -> (w951:string)
            n1145 = call-poly "FeedbackDecode_VariablesToString.vi"("Format"="%0.0f", "ValueIn"=w947, "FieldName"="NIPTime" ("Key Word")) -> ("StringOut"=w939:string)  [unwired: 4 in]
            n1146 = local read "EventParamsFID"() -> (w950:refnum<file>)
            n1147 = local read "DecodeClust"() -> (w955:T5)
            n1148 = Concatenate Strings(w951, w938, w939) -> (w949:string)
            n1149 = call "FeedbackDecode_WriteTextEOL.vi"("text"=w949, "refnum in"=w950) -> ()  [unwired: 8 in, 2 out]
            n1150 = Bundle By Name(cluster=w955, "EventStr"=w949) -> (w948:T5)
            n1151 = call "FeedbackDecode_MLComCtrl.vi"("DecodeClustIn"=w948, "Mode"=T19."SendEvent") -> ()  [unwired: 6 in, 4 out]
          }
          event Value Change {
            n1152 = event-data() -> ("NewVal"=w963:bool)  [unwired: 1 in, 5 out]
            n1153 = case shown="True" w963 {
              frame False {
                n1154 = local read "LoopCnt"() -> (w975:u64)
                n1155 = local read "NIPTime"() -> (w969:dbl)
                n1156 = Format Into String(w975) -> (resulting string=w965:string)  [unwired: 3 in, 1 out]
                n1157 = Concatenate Strings("DisableLog10:SS.EventID=" ("string"), w965) -> (w974:string)
                n1158 = local read "EventParamsFID"() -> (w972:refnum<file>)
                n1159 = call-poly "FeedbackDecode_VariablesToString.vi"("Format"="%0.0f", "ValueIn"=w969, "FieldName"="NIPTime" ("Key Word")) -> ("StringOut"=w966:string)  [unwired: 4 in]
                n1160 = local read "DecodeClust"() -> (w978:T5)
                n1161 = Concatenate Strings(w974, ";SS.Log10=0;" ("EventStr"), w966) -> (w971:string)
                n1162 = call "FeedbackDecode_WriteTextEOL.vi"("text"=w971, "refnum in"=w972) -> ()  [unwired: 8 in, 2 out]
                n1163 = Bundle By Name(cluster=w978, "EventStr"=w971) -> (w970:T5)
                n1164 = call "FeedbackDecode_MLComCtrl.vi"("DecodeClustIn"=w970, "Mode"=T19."SendEvent") -> ()  [unwired: 6 in, 4 out]
              }
              frame True {
                n1165 = local read "LoopCnt"() -> (w990:u64)
                n1166 = local read "NIPTime"() -> (w983:dbl)
                n1167 = Format Into String(w990) -> (resulting string=w979:string)  [unwired: 3 in, 1 out]
                n1168 = Concatenate Strings("EnableLog10:SS.EventID=" ("string"), w979) -> (w989:string)
                n1169 = local read "EventParamsFID"() -> (w987:refnum<file>)
                n1170 = call-poly "FeedbackDecode_VariablesToString.vi"("Format"="%0.0f", "ValueIn"=w983, "FieldName"="NIPTime" ("Key Word")) -> ("StringOut"=w980:string)  [unwired: 4 in]
                n1171 = local read "DecodeClust"() -> (w985:T5)
                n1172 = Concatenate Strings(w989, ";SS.Log10=1;" ("EventStr"), w980) -> (w986:string)
                n1173 = call "FeedbackDecode_WriteTextEOL.vi"("text"=w986, "refnum in"=w987) -> ()  [unwired: 8 in, 2 out]
                n1174 = Bundle By Name(cluster=w985, "EventStr"=w986) -> (w984:T5)
                n1175 = call "FeedbackDecode_MLComCtrl.vi"("DecodeClustIn"=w984, "Mode"=T19."SendEvent") -> ()  [unwired: 6 in, 4 out]
              }
            }
          }
          event Value Change {
            n1176 = event-data() -> ("NewVal"=w993:bool)  [unwired: 1 in, 5 out]
            n1177 = case shown="True" w993 {
              frame False {
                n1178 = local read "LoopCnt"() -> (w1005:u64)
                n1179 = local read "NIPTime"() -> (w999:dbl)
                n1180 = Format Into String(w1005) -> (resulting string=w995:string)  [unwired: 3 in, 1 out]
                n1181 = Concatenate Strings("DisableReTrain:SS.EventID=" ("string"), w995) -> (w1004:string)
                n1182 = call-poly "FeedbackDecode_VariablesToString.vi"("Format"="%0.0f", "ValueIn"=w999, "FieldName"="NIPTime" ("Key Word")) -> ("StringOut"=w996:string)  [unwired: 4 in]
                n1183 = local read "EventParamsFID"() -> (w1002:refnum<file>)
                n1184 = local read "DecodeClust"() -> (w1008:T5)
                n1185 = Concatenate Strings(w1004, ";SS.ReTrain=0;" ("EventStr"), w996) -> (w1001:string)
                n1186 = call "FeedbackDecode_WriteTextEOL.vi"("text"=w1001, "refnum in"=w1002) -> ()  [unwired: 8 in, 2 out]
                n1187 = Bundle By Name(cluster=w1008, "EventStr"=w1001) -> (w1000:T5)
                n1188 = call "FeedbackDecode_MLComCtrl.vi"("DecodeClustIn"=w1000, "Mode"=T19."SendEvent") -> ()  [unwired: 6 in, 4 out]
              }
              frame True {
                n1189 = local read "LoopCnt"() -> (w1019:u64)
                n1190 = local read "NIPTime"() -> (w1013:dbl)
                n1191 = Format Into String(w1019) -> (resulting string=w1009:string)  [unwired: 3 in, 1 out]
                n1192 = Concatenate Strings("EnableReTrain:SS.EventID=" ("string"), w1009) -> (w1018:string)
                n1193 = local read "EventParamsFID"() -> (w1016:refnum<file>)
                n1194 = call-poly "FeedbackDecode_VariablesToString.vi"("Format"="%0.0f", "ValueIn"=w1013, "FieldName"="NIPTime" ("Key Word")) -> ("StringOut"=w1010:string)  [unwired: 4 in]
                n1195 = local read "DecodeClust"() -> (w1022:T5)
                n1196 = Concatenate Strings(w1018, ";SS.ReTrain=1;" ("EventStr"), w1010) -> (w1015:string)
                n1197 = call "FeedbackDecode_WriteTextEOL.vi"("text"=w1015, "refnum in"=w1016) -> ()  [unwired: 8 in, 2 out]
                n1198 = Bundle By Name(cluster=w1022, "EventStr"=w1015) -> (w1014:T5)
                n1199 = call "FeedbackDecode_MLComCtrl.vi"("DecodeClustIn"=w1014, "Mode"=T19."SendEvent") -> ()  [unwired: 6 in, 4 out]
              }
            }
          }
          event Value Change {
            n1200 = event-data() -> ("NewVal"=w1024:dbl)  [unwired: 1 in, 5 out]
            n1201 = local read "LoopCnt"() -> (w1037:u64)
            n1202 = call-poly "FeedbackDecode_VariablesToString.vi"("Format"="%0.5f", "ValueIn"=w1024, "FieldName"="FreeParam") -> ("StringOut"=w1023:string)  [unwired: 4 in]
            n1203 = local read "NIPTime"() -> (w1031:dbl)
            n1204 = Format Into String(w1037) -> (resulting string=w1027:string)  [unwired: 3 in, 1 out]
            n1205 = Concatenate Strings("UpdateFreeParam:SS.EventID=" ("string"), w1027) -> (w1036:string)
            n1206 = local read "EventParamsFID"() -> (w1034:refnum<file>)
            n1207 = call-poly "FeedbackDecode_VariablesToString.vi"("Format"="%0.0f", "ValueIn"=w1031, "FieldName"="NIPTime" ("Key Word")) -> ("StringOut"=w1028:string)  [unwired: 4 in]
            n1208 = local read "DecodeClust"() -> (w1040:T5)
            n1209 = Concatenate Strings(w1036, ";" ("EventStr"), w1023, w1028) -> (w1033:string)
            n1210 = call "FeedbackDecode_WriteTextEOL.vi"("text"=w1033, "refnum in"=w1034) -> ()  [unwired: 8 in, 2 out]
            n1211 = Bundle By Name(cluster=w1040, "EventStr"=w1033) -> (w1032:T5)
            n1212 = call "FeedbackDecode_MLComCtrl.vi"("DecodeClustIn"=w1032, "Mode"=T19."SendEvent") -> ()  [unwired: 6 in, 4 out]
          }
          event Value Change {
            n1213 = event-data() -> ("NewVal"=w1043:dbl)  [unwired: 1 in, 5 out]
            n1214 = local read "LoopCnt"() -> (w1056:u64)
            n1215 = call-poly "FeedbackDecode_VariablesToString.vi"("Format"="%0.5f", "ValueIn"=w1043, "FieldName"="GoalNoise") -> ("StringOut"=w1042:string)  [unwired: 4 in]
            n1216 = local read "NIPTime"() -> (w1050:dbl)
            n1217 = Format Into String(w1056) -> (resulting string=w1046:string)  [unwired: 3 in, 1 out]
            n1218 = Concatenate Strings("UpdateGoalNoise:SS.EventID=" ("string"), w1046) -> (w1055:string)
            n1219 = local read "EventParamsFID"() -> (w1053:refnum<file>)
            n1220 = call-poly "FeedbackDecode_VariablesToString.vi"("Format"="%0.0f", "ValueIn"=w1050, "FieldName"="NIPTime" ("Key Word")) -> ("StringOut"=w1047:string)  [unwired: 4 in]
            n1221 = local read "DecodeClust"() -> (w1059:T5)
            n1222 = Concatenate Strings(w1055, ";" ("EventStr"), w1042, w1047) -> (w1052:string)
            n1223 = call "FeedbackDecode_WriteTextEOL.vi"("text"=w1052, "refnum in"=w1053) -> ()  [unwired: 8 in, 2 out]
            n1224 = Bundle By Name(cluster=w1059, "EventStr"=w1052) -> (w1051:T5)
            n1225 = call "FeedbackDecode_MLComCtrl.vi"("DecodeClustIn"=w1051, "Mode"=T19."SendEvent") -> ()  [unwired: 6 in, 4 out]
          }
          event "OffSet": Value Change {
            n1226 = event-data() -> ("NewVal"=w1062:dbl)  [unwired: 1 in, 5 out]
            n1227 = global write "FeedbackDecode_Globals.vi" "FD_ForceOffset"(w1062) -> ()
          }
          event Value Change {
            n1228 = event-data() -> ("NewVal"=w1064:bool)  [unwired: 1 in, 5 out]
            n1229 = case shown="True" w1064 {
              frame False {
              }
              frame True {
                n1230 = local read "DecodeClust"() -> (w1069:T5)
                n1231 = Unbundle By Name(w1069) -> ("CompID.ML.Name"=w1068:string, "DataFolder"=w1067:string, "DataDir"=w1065:string, "NumComp"=w1066:enum16{"1 Computer", "2 Computers"})
                n1232 = case shown="\"1 Computer\"" w1066 {
                  tunnel: w1069 -> [w1089 w1118]
                  tunnel: w1068 -> [w1073 _]
                  tunnel: w1067 -> [w1072 w1102]
                  tunnel: w1065 -> [_ w1099]
                  frame "2 Computers", Default {
                    n1233 = call "FeedbackDecode_CopyRemoteFiles.vi"("DataFolder"=w1072, "CompName"=w1073, "Mode"=enum16{"Decode", "Encode"}."Decode") -> ("OrigName"=w1070:string, "MLName"=w1096:string)  [unwired: 1 in]
                    n1234 = local read "LoopCnt"() -> (w1086:u64)
                    n1235 = local read "NIPTime"() -> (w1090:dbl)
                    n1236 = String To Path(string=w1096) -> (path=w1095:path)
                    n1237 = Strip Path(path=w1095) -> (name=w1097:string)  [unwired: 1 out]
                    n1238 = Format Into String(w1086) -> (resulting string=w1098:string)  [unwired: 3 in, 1 out]
                    n1239 = call-poly "FeedbackDecode_VariablesToString.vi"("Format"="%0.0f", "ValueIn"=w1090, "FieldName"="NIPTime" ("Key Word")) -> ("StringOut"=w1093:string)  [unwired: 4 in]
                    n1240 = Concatenate Strings("SS.TrainFileLV='" ("string"), w1096, "';" ("string")) -> (w1080:string)
                    n1241 = Concatenate Strings("LoadTrainFile:SS.EventID=" ("string"), w1098) -> (w1087:string)
                    n1242 = Concatenate Strings("SS.TrainFileOrig='" ("string"), w1070, "';" ("string"), w1093) -> (w1076:string)
                    n1243 = Concatenate Strings(w1087, ";", w1080) -> (w1079:string)
                    n1244 = Concatenate Strings(w1079, w1076) -> (w1074:string)
                    n1245 = Bundle By Name(cluster=w1089, "KDFFile"=w1097, "EventStr"=w1079) -> (w1088:T5)
                    n1246 = local read "EventParamsFID"() -> (w1075:refnum<file>)
                    n1247 = call "FeedbackDecode_WriteTextEOL.vi"("text"=w1074, "refnum in"=w1075) -> ()  [unwired: 8 in, 2 out]
                    n1248 = call "FeedbackDecode_MLComCtrl.vi"("DecodeClustIn"=w1088, "Mode"=T19."SendEvent") -> ("DecodeClustOut"=w1094:T5)  [unwired: 6 in, 3 out]
                    n1249 = local write "DecodeClust"(w1094) -> ()
                  }
                  frame "1 Computer" {
                    n1250 = call "FeedbackDecode_CopyLocalFiles.vi"("DataFolder"=w1102, "DataDir"=w1099, "Mode"=enum16{"Decode", "Encode"}."Decode") -> ("OrigName"=w1100:string, "MLName"=w1125:string)  [unwired: 1 in]
                    n1251 = local read "LoopCnt"() -> (w1115:u64)
                    n1252 = local read "NIPTime"() -> (w1119:dbl)
                    n1253 = String To Path(string=w1125) -> (path=w1124:path)
                    n1254 = Strip Path(path=w1124) -> (name=w1126:string)  [unwired: 1 out]
                    n1255 = Format Into String(w1115) -> (resulting string=w1127:string)  [unwired: 3 in, 1 out]
                    n1256 = call-poly "FeedbackDecode_VariablesToString.vi"("Format"="%0.0f", "ValueIn"=w1119, "FieldName"="NIPTime" ("Key Word")) -> ("StringOut"=w1122:string)  [unwired: 4 in]
                    n1257 = Concatenate Strings("SS.TrainFileLV='" ("string"), w1125, "';" ("string")) -> (w1109:string)
                    n1258 = Concatenate Strings("LoadTrainFile:SS.EventID=" ("string"), w1127) -> (w1116:string)
                    n1259 = Concatenate Strings("SS.TrainFileOrig='" ("string"), w1100, "';" ("string"), w1122) -> (w1105:string)
                    n1260 = Concatenate Strings(w1116, ";", w1109) -> (w1108:string)
                    n1261 = Concatenate Strings(w1108, w1105) -> (w1103:string)
                    n1262 = Bundle By Name(cluster=w1118, "KDFFile"=w1126, "EventStr"=w1108) -> (w1117:T5)
                    n1263 = local read "EventParamsFID"() -> (w1104:refnum<file>)
                    n1264 = call "FeedbackDecode_WriteTextEOL.vi"("text"=w1103, "refnum in"=w1104) -> ()  [unwired: 8 in, 2 out]
                    n1265 = call "FeedbackDecode_MLComCtrl.vi"("DecodeClustIn"=w1117, "Mode"=T19."SendEvent") -> ("DecodeClustOut"=w1123:T5)  [unwired: 6 in, 3 out]
                    n1266 = local write "DecodeClust"(w1123) -> ()
                  }
                }
              }
            }
          }
          event Value Change {
            n1267 = event-data() -> ("NewVal"=w1129:bool)  [unwired: 1 in, 5 out]
            n1268 = case shown="True" w1129 {
              frame False {
                n1269 = local read "LoopCnt"() -> (w1140:u64)
                n1270 = local read "NIPTime"() -> (w1134:dbl)
                n1271 = Format Into String(w1140) -> (resulting string=w1130:string)  [unwired: 3 in, 1 out]
                n1272 = Concatenate Strings("DisableNIPSpikes:SS.EventID=" ("string"), w1130) -> (w1139:string)
                n1273 = local read "EventParamsFID"() -> (w1137:refnum<file>)
                n1274 = call-poly "FeedbackDecode_VariablesToString.vi"("Format"="%0.0f", "ValueIn"=w1134, "FieldName"="NIPTime" ("Key Word")) -> ("StringOut"=w1131:string)  [unwired: 4 in]
                n1275 = local read "DecodeClust"() -> (w1143:T5)
                n1276 = Concatenate Strings(w1139, ";SS.NIPSpikes=0;" ("EventStr"), w1131) -> (w1136:string)
                n1277 = call "FeedbackDecode_WriteTextEOL.vi"("text"=w1136, "refnum in"=w1137) -> ()  [unwired: 8 in, 2 out]
                n1278 = Bundle By Name(cluster=w1143, "EventStr"=w1136) -> (w1135:T5)
                n1279 = call "FeedbackDecode_MLComCtrl.vi"("DecodeClustIn"=w1135, "Mode"=T19."SendEvent") -> ()  [unwired: 6 in, 4 out]
              }
              frame True {
                n1280 = local read "LoopCnt"() -> (w1154:u64)
                n1281 = local read "NIPTime"() -> (w1148:dbl)
                n1282 = Format Into String(w1154) -> (resulting string=w1144:string)  [unwired: 3 in, 1 out]
                n1283 = Concatenate Strings("EnableNIPSpikes:SS.EventID=" ("string"), w1144) -> (w1153:string)
                n1284 = call-poly "FeedbackDecode_VariablesToString.vi"("Format"="%0.0f", "ValueIn"=w1148, "FieldName"="NIPTime" ("Key Word")) -> ("StringOut"=w1145:string)  [unwired: 4 in]
                n1285 = local read "EventParamsFID"() -> (w1151:refnum<file>)
                n1286 = local read "DecodeClust"() -> (w1157:T5)
                n1287 = Concatenate Strings(w1153, ";SS.NIPSpikes=1;" ("EventStr"), w1145) -> (w1150:string)
                n1288 = call "FeedbackDecode_WriteTextEOL.vi"("text"=w1150, "refnum in"=w1151) -> ()  [unwired: 8 in, 2 out]
                n1289 = Bundle By Name(cluster=w1157, "EventStr"=w1150) -> (w1149:T5)
                n1290 = call "FeedbackDecode_MLComCtrl.vi"("DecodeClustIn"=w1149, "Mode"=T19."SendEvent") -> ()  [unwired: 6 in, 4 out]
              }
            }
          }
          event Value Change {
            n1291 = event-data() -> ("NewVal"=w1159:bool)  [unwired: 1 in, 5 out]
            n1292 = case shown="True" w1159 {
              frame False {
              }
              frame True {
                n1293 = local read "DecodeClust"() -> (w1187:T5)
                n1294 = Unbundle By Name(w1187) -> ("AutoPopType"=w1163:enum16{"Standard", "Stepwise", "Gram"}, "AutoThresh"=w1184:dbl, "BadUEAElects"=w1177:dbl[], "BadEMGChans"=w1181:dbl[])
                n1295 = Format Into String(w1163) -> (resulting string=w1161:string)  [unwired: 3 in, 1 out]
                n1296 = local read "LoopCnt"() -> (w1173:u64)
                n1297 = call-poly "FeedbackDecode_VariablesToString.vi"("ValueIn"=w1161, "FieldName"="AutoPopType" ("Key Word")) -> ("StringOut"=w1160:string)  [unwired: 5 in]
                n1298 = call-poly "FeedbackDecode_VariablesToString.vi"("ValueIn"=w1184, "FieldName"="AutoThresh") -> ("StringOut"=w1180:string)  [unwired: 5 in]
                n1299 = call-poly "FeedbackDecode_VariablesToString.vi"("ValueIn"=w1177, "FieldName"="BadUEAElects") -> ("StringOut"=w1179:string)  [unwired: 5 in]
                n1300 = call-poly "FeedbackDecode_VariablesToString.vi"("ValueIn"=w1181, "FieldName"="BadEMGChans") -> ("StringOut"=w1178:string)  [unwired: 5 in]
                n1301 = Format Into String(w1173) -> (resulting string=w1164:string)  [unwired: 3 in, 1 out]
